vi "MotionProfiles_Init.vi"(4 "Wheel_Diameter (in)":dbl=4.0, 6 "MP_Frame_Rate_(ms)":i32=5, 7 "Encoder_CPR_4x":dbl=240.0, 8 "error in (no error)":errorcluster, 9 "CSV File Path":path=path "/home/lvuser/mp.csv", 10 "PhoenixMotorControlDevRef":T1={"DeviceStatus"={"status"=FALSE, "code"=0, "source"=""}, "Type"=enum."PWM", "PWM"={"PWM Channel"=enum."Invalid", "DeadBand"={"Name"="", "maxPositivePwm"=0, "minPositivePwm"=0, "centerPwm"=0, "maxNegativePwm"=0, "minNegativePwm"=0, "angularRange"=0}}, "CAN"={"Device Number"=0, "SetOutput VI Ref"=variant(refnum<vi> refnum), "GetOutput VI Ref"=variant(refnum<vi> refnum), "Enable VI Ref"=variant(refnum<vi> refnum), "Disable VI Ref"=variant(refnum<vi> refnum), "Data"=variant}, "Invert"=FALSE, "DIO PWM"={"PWM \"Enable\" Channel"=enum."Invalid", "DIOChannel"=enum."Invalid", "PWM Rate"=0.0}}, 11 "MotionProfiles in":refnum<class "MotionProfiles.lvclass">) -> (0 "error out":errorcluster, 3 "MotionProfiles out":refnum<class "MotionProfiles.lvclass">)   [LabVIEW 2018, in "MotionProfiles.lvclass"]
uses:
  MotionProfiles.lvclass
  <vilib>/Rock Robotics/WPI/MotorControl/WPI_MotorControlDeviceRef.ctl
  <vilib>/Rock Robotics/WPI/MotorControl/WPI_MotorControlType.ctl
  <vilib>/Rock Robotics/SystemInterfaces/DIO/FPGA_DIOPWMChannel.ctl
  <vilib>/Rock Robotics/WPI/PWM/WPI_PWMDeadband.ctl
  <vilib>/Rock Robotics/SystemInterfaces/DIO/FPGA_DIOChannel.ctl
  MotionProfile_InternalStateEnum.ctl
  MotionProfile_TalonSetValueEnum.ctl
  MotionProfile_TrajectoryPoint.ctl
  MotionProfiles.lvclass/MotionProfiles.ctl
  <vilib>/Utility/file.llb/Read Delimited Spreadsheet (DBL).vi
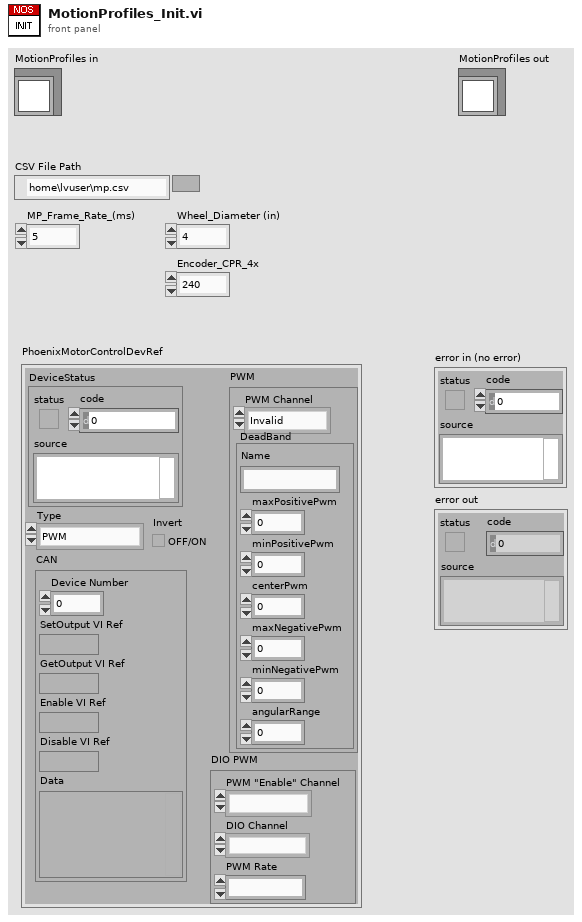
[diagram p1: front panel]
types:
  T1 = typedef "WPI_MotorControlDeviceRef.ctl" = cluster{"DeviceStatus":errorcluster, "Type":T2, "PWM":cluster{"PWM Channel":T3, "DeadBand":T4}, "CAN":cluster{"Device Number":u8, "SetOutput VI Ref":variant, "GetOutput VI Ref":variant, "Enable VI Ref":variant, "Disable VI Ref":variant, "Data":variant}, "Invert":bool, "DIO PWM":cluster{"PWM \"Enable\" Channel":T3, "DIOChannel":T5, "PWM Rate":dbl}}
  T2 = typedef "WPI_MotorControlType.ctl" = enum16{"PWM", "CAN", "DIO PWM"}
  T3 = typedef "FPGA_DIOPWMChannel.ctl" = enum8{"PWM 0", "PWM 1", "PWM 2", "PWM 3", "PWM 4", "PWM 5", "PWM 6", "PWM 7", "PWM 8", "PWM 9", "PWM MXP 0", "PWM MXP 1", "PWM MXP 2", "PWM MXP 3", "PWM MXP 4", "PWM MXP 5", "PWM MXP 6", "PWM MXP 7", "PWM MXP 8", "PWM MXP 9", "Invalid"}
  T4 = typedef "WPI_PWMDeadband.ctl" = cluster{"Name":string, "maxPositivePwm":i32, "minPositivePwm":i32, "centerPwm":i32, "maxNegativePwm":i32, "minNegativePwm":i32, "angularRange":u16}
  T5 = typedef "FPGA_DIOChannel.ctl" = enum8{"DIO 0", "DIO 1", "DIO 2", "DIO 3", "DIO 4", "DIO 5", "DIO 6", "DIO 7", "DIO 8", "DIO 9", "DIO MXP 0", "DIO MXP 1", "DIO MXP 2", "DIO MXP 3", "DIO MXP 4", "DIO MXP 5", "DIO MXP 6", "DIO MXP 7", "DIO MXP 8", "DIO MXP 9", "DIO MXP 10", "DIO MXP 11", "DIO MXP 12", "DIO MXP 13", "DIO MXP 14", "DIO MXP 15", "SPI Port CS1", "SPI Port CS2", "SPI Port CS3", "SPI Port MISO", "SPI Port MOSI", "Invalid"}
  T6 = typedef "MotionProfiles.lvclass/MotionProfile_TrajectoryPoint.ctl" = cluster{"Duration (ms)":u8, "Velocity (u/100ms)":dbl, "Position (units)":dbl, "Profile Slot Select":u8, "Is Last":bool, "Velocity Only":bool, "Zero Position":bool, "Compress Code":u8, "Same Velocity":i32, "Delta Position":i32, "Count":u8, "Invert Motors?":bool}
  T7 = typedef "MotionProfiles.lvclass/MotionProfile_TalonSetValueEnum.ctl" = enum16{"Disable", "Enable", "Hold"}
  T8 = typedef "MotionProfiles.lvclass/MotionProfile_InternalStateEnum.ctl" = enum16{"Nothing", "Send Points to Talon", "Run Profile"}
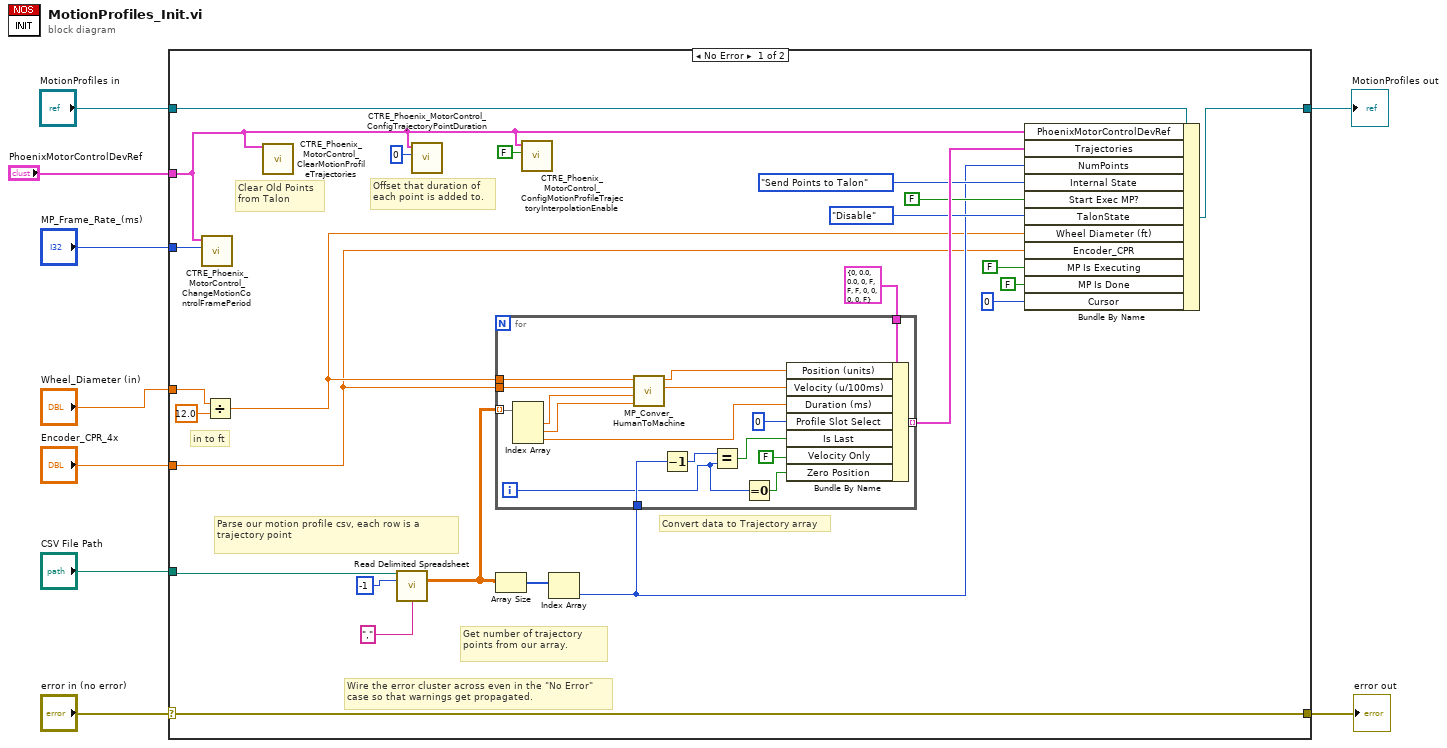
[diagram p0: block diagram]
diagram:
  n1 = case shown="No Error" "error in (no error)" {
    selector: "error in (no error)" -> [w34 w53]
    tunnel: [w34 w53] -> w8
    tunnel: [w33 w52] -> w6
    tunnel: "MotionProfiles in" -> [w21 w52]
    tunnel: "PhoenixMotorControlDevRef" -> [w11 _]
    tunnel: "CSV File Path" -> [w31 _]
    tunnel: "MP_Frame_Rate_(ms)" -> [w20 _]
    tunnel: "Wheel_Diameter (in)" -> [w26 _]
    tunnel: "Encoder_CPR_4x" -> [w12 _]
    frame No Error {
      # "Offset that duration of \neach point is added to."
      # "in to ft"
      # "Clear Old Points\nfrom Talon"
      # "Convert data to Trajectory array"
      # "Get number of trajectory points from our array."
      # "Parse our motion profile csv, each row is a trajectory point"
      # "Wire the error cluster across even in the \"No Error\"\ncase so that warnings get propagated."
      n2 = call <vilib>:"CTRE_Phoenix_MotorControl_ChangeMotionControlFramePeriod.vi"("periodMs"=w20, "PhoenixMotorControlDevRef"=w11) -> ()  [unwired: 8 in, 2 out]
      n3 = Divide(x=w26, y=12.0) -> (x/y=w17:dbl)
      n4 = call <vilib>:"CTRE_Phoenix_MotorControl_ClearMotionProfileTrajectories.vi"("PhoenixMotorControlDevRef"=w11) -> ()  [unwired: 13 in, 2 out]
      n5 = call-poly <vilib>:"Read Delimited Spreadsheet.vi"("file path (dialog if empty)"=w31, "number of rows (all:-1)"=-1, "delimiter (\\t)"="," ("delimiter (\\t)")) -> ("all rows"=w23:dbl[][])  [unwired: 7 in, 5 out]
      n6 = call <vilib>:"CTRE_Phoenix_MotorControl_ConfigTrajectoryPointDuration.vi"("durationMs"=0, "PhoenixMotorControlDevRef"=w11) -> ()  [unwired: 8 in, 2 out]
      n7 = Array Size(array=w23) -> (size(s)=w22:i32[])
      n8 = call <vilib>:"CTRE_Phoenix_MotorControl_ConfigMotionProfileTrajectoryInterpolationEnable.vi"("enable?"=FALSE, "PhoenixMotorControlDevRef"=w11) -> ()  [unwired: 8 in, 2 out]
      n9 = Index Array(array=w22) -> (element=w18:i32)  [unwired: 1 in]
      n10 = for {
        tunnel: [w49] -> w30 mode=indexing
        tunnel: w23 -> [w47] mode=indexing
        tunnel: T6 {"Duration (ms)"=0, "Velocity (u/100ms)"=0.0, "Position (units)"=0.0, "Profile Slot Select"=0, "Is Last"=FALSE, "Velocity Only"=FALSE, "Zero Position"=FALSE, "Compress Code"=0, "Same Velocity"=0, "Delta Position"=0, "Count"=0, "Invert Motors?"=FALSE} ("Motion Profile Trajectory Point") -> [w46]
        tunnel: w18 -> [w42]
        tunnel: w17 -> [w41]
        tunnel: w12 -> [w40]
        i -> [w36]
        n11 = Index Array(array=w47) -> (element #1=w39:dbl, element #2=w38:dbl, element #3=w45:dbl)  [unwired: 3 in]
        n12 = call "MP_Conver_HumanToMachine.vi"("Vel_In (ft/s)"=w38, "Pos_In (ft)"=w39, "CPR"=w40, "Diameter (ft)"=w41) -> ("Vel_Out (u/100ms)"=w37:dbl, "Pos_Out (u)"=w35:dbl)  [unwired: 4 in]
        n13 = Decrement(x=w42) -> (x-1=w43:i32)
        n14 = Equal?(x=w43, y=w36) -> (x = y?=w44:bool)
        n15 = Equal To 0?(x=w36) -> (x = 0?=w50:bool)
        n16 = Bundle By Name(cluster=w46, "Position (units)"=w35, "Velocity (u/100ms)"=w37, "Duration (ms)"=w45, "Profile Slot Select"=u8 0, "Is Last"=w44, "Velocity Only"=FALSE, "Zero Position"=w50) -> (w49:T6)
      }
      n17 = Bundle By Name(cluster=w21, "PhoenixMotorControlDevRef"=w11, "Trajectories"=w30, "NumPoints"=w18, "Internal State"=MotionProfile_InternalStateEnum."Send Points to Talon", "Start Exec MP?"=FALSE, "TalonState"=MotionProfile_TalonSetValueEnum."Disable" ("TalonSetValue"), "Wheel Diameter (ft)"=w17, "Encoder_CPR"=w12, "MP Is Executing"=FALSE, "MP Is Done"=FALSE, "Cursor"=u32 0) -> (w33:refnum<class "MotionProfiles.lvclass">)
    }
    frame Error {
    }
  }
  "error out" <- w8
  "MotionProfiles out" <- w6
